vi "test8-UserLog_Queue.vi"(8 "error in (no error)":errorcluster, 11 "TestCase in":refnum<class "testcase-CSMGlobalLog.lvclass">) -> (0 "error out":errorcluster, 3 "TestCase out":refnum<class "testcase-CSMGlobalLog.lvclass">)   [LabVIEW 2017, in "testcase-CSMGlobalLog.lvclass"]
uses:
  testcase-CSMGlobalLog.lvclass
  testcase-CSMGlobalLog.lvclass/testcase-CSMGlobalLog.ctl
  ed57623f-cc02-4141-adee-02d92d4e7552.vi
  src/user.lib/_NEVSTOP/Communicable State Machine(CSM)/_Support/GlobalEvent/GEvt-Generate with Rule Check.vi
  src/user.lib/_NEVSTOP/Communicable State Machine(CSM)/AdvanceAPI/CSM - Convert Error to Argument.vi
  src/user.lib/_NEVSTOP/Communicable State Machine(CSM)/AdvanceAPI/CSM - Make String Arguments Safe.vi
  src/user.lib/_NEVSTOP/Communicable State Machine(CSM)/AdvanceAPI/CSM - Keywords.vi
  src/user.lib/_NEVSTOP/Communicable State Machine(CSM)/_Support/GlobalEvent/Cache-GEvt Refs.vi
  src/user.lib/_NEVSTOP/Communicable State Machine(CSM)/_Support/GlobalEvent/LogFilter/LogFilter - Check.vi
  src/user.lib/_NEVSTOP/Communicable State Machine(CSM)/_Support/GlobalEvent/LogFilter/LogFilter.lvclass
  <vilib>/addons/_JKI Toolkits/VI Tester/TestCase.llb/TestCase.lvclass
  src/user.lib/_NEVSTOP/Communicable State Machine(CSM)/Communicable State Machine.lvlib
  src/user.lib/_NEVSTOP/Communicable State Machine(CSM)/Utility/Periodic String Filter Setting.ctl
  C:/Program Files (x86)/National Instruments/LabVIEW 2017/vi.lib/addons/_JKI Toolkits/VI Tester/TestCase.llb/TestCase.lvclass
panel:
  out "String cache total":string
  out "error out 2":errorcluster
  out "LoopCount":i32
  out "String Cache Each Loop":string
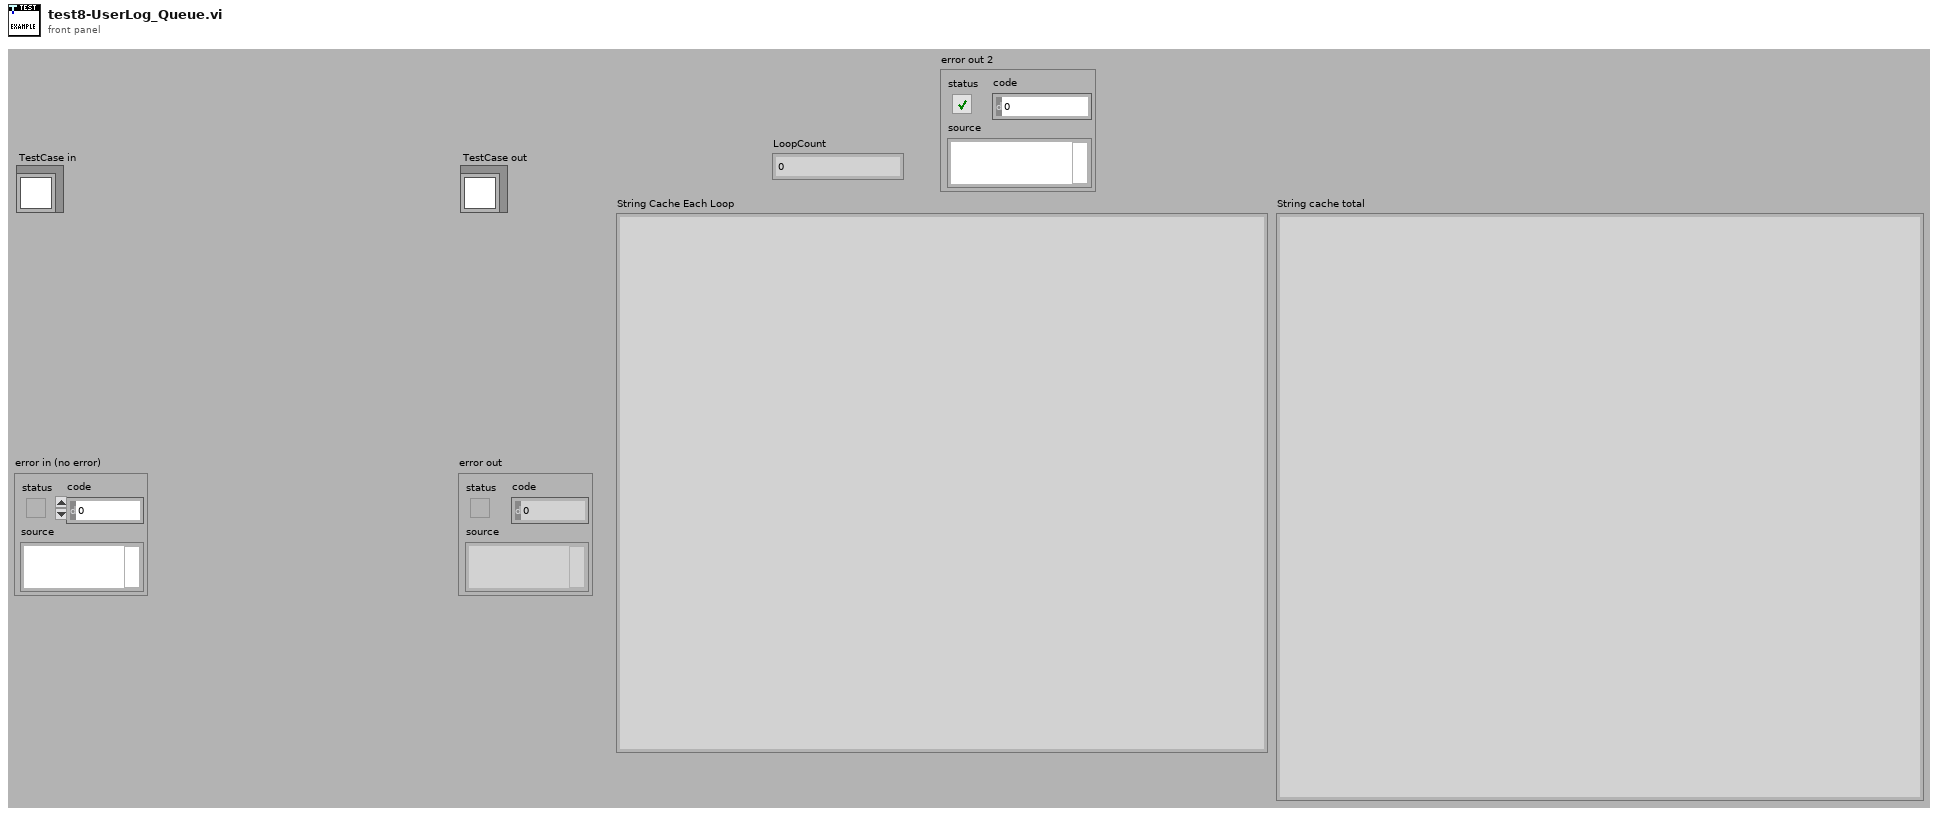
[diagram p1: front panel]
types:
  T1 = typedef "Communicable State Machine.lvlib/Periodic String Filter Setting.ctl" = cluster{"threashold(#/s)":dbl, "Check Peroid(s)":dbl}
  T2 = typedef "Communicable State Machine.lvlib/_CSM_GlobalLog_MSG.ctl" = cluster{"Name (\"\" to Use UUID)":string, "Current State":string, "Arguments":string, "Source Message":T3, "Source Module":string, "Complete(T)/Start(F)":bool, "LogType":T4, "Time Stamp":timestamp}
  T3 = typedef "Communicable State Machine.lvlib/_CSM_Response Source Message.ctl" = cluster{"‘State":string, "’Arguments":string, "’Error":errorcluster}
  T4 = typedef "Communicable State Machine.lvlib/_CSM_GlobalLog_MSG_TYPE.ctl" = enum16{"User Log", "State Change", "Status", "Interrupt", "Register", "Unregister", "Error Log", "Module Created", "Module Destroyed"}
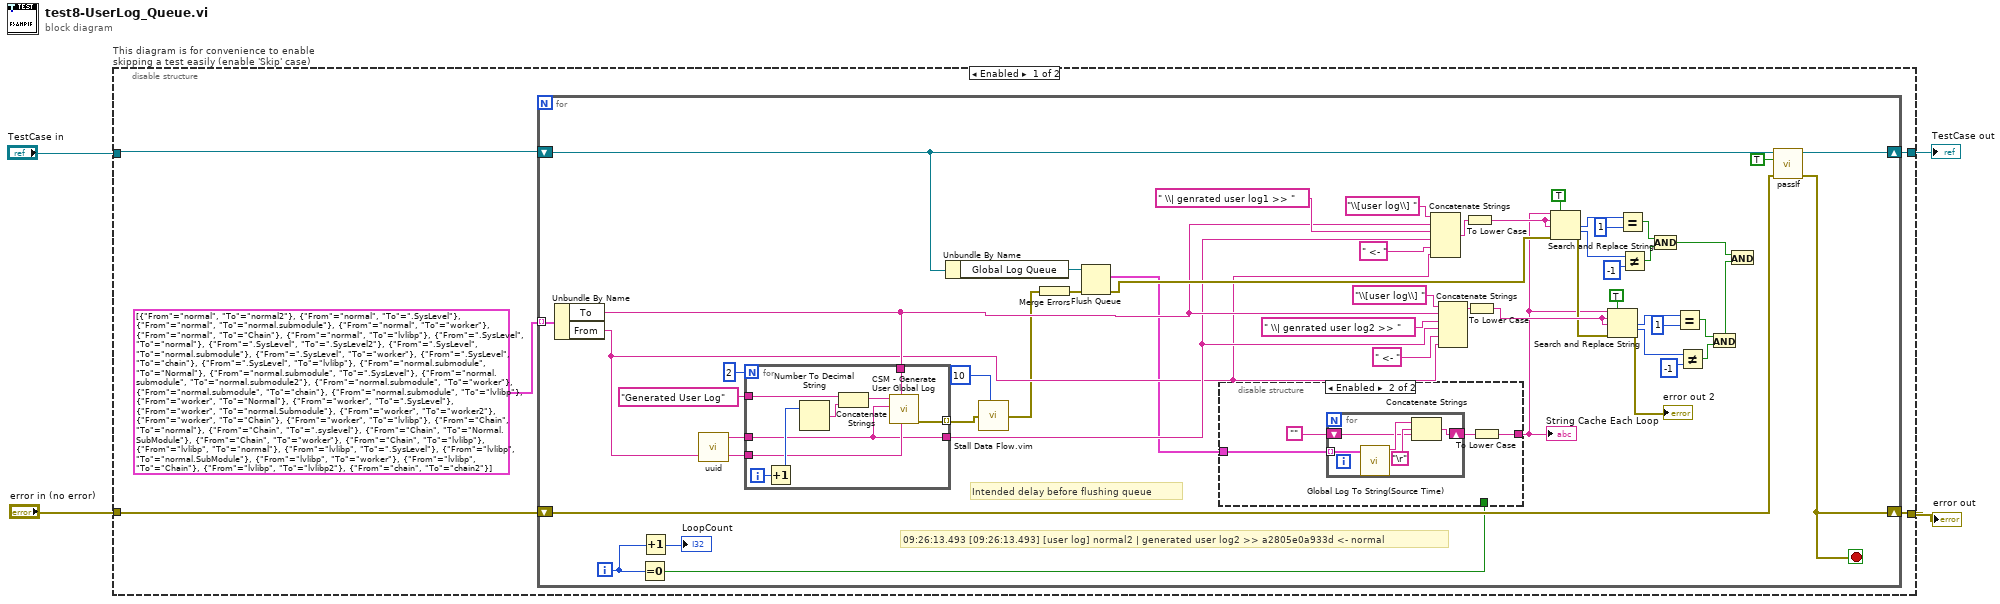
[diagram p0: block diagram]
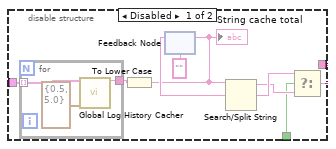
[diagram p2: hidden frame]
diagram:
  n1 = disable-structure "This diagram is for convenience to enable skipping a test easily (enable 'Skip' case)" shown="Enabled" {
    disable-tunnel: "TestCase in" -> [w6 w94]
    disable-tunnel: [w8 w92] -> w1
    disable-tunnel: [w9 w93] -> w3
    disable-tunnel: "error in (no error)" -> [w7 w91]
    frame Enabled {
      n2 = for {
        shift-right: [w35] -> w9
        shift-left: w7 -> [w58]
        shift-right: [w60] -> w8
        shift-left: w6 -> [w34]
        tunnel: cluster{"From":string, "To":string}[] [{"From"="normal", "To"="normal2"}, {"From"="normal", "To"=".SysLevel"}, {"From"="normal", "To"="normal.submodule"}, {"From"="normal", "To"="worker"}, {"From"="normal", "To"="Chain"}, {"From"="normal", "To"="lvlibp"}, {"From"=".SysLevel", "To"="normal"}, {"From"=".SysLevel", "To"=".SysLevel2"}, {"From"=".SysLevel", "To"="normal.submodule"}, {"From"=".SysLevel", "To"="worker"}, {"From"=".SysLevel", "To"="chain"}, {"From"=".SysLevel", "To"="lvlibp"}, {"From"="normal.submodule", "To"="Normal"}, {"From"="normal.submodule", "To"=".SysLevel"}, {"From"="normal.submodule", "To"="normal.submodule2"}, {"From"="normal.submodule", "To"="worker"}, {"From"="normal.submodule", "To"="chain"}, {"From"="normal.submodule", "To"="lvlibp"}, {"From"="worker", "To"="Normal"}, {"From"="worker", "To"=".SysLevel"}, {"From"="worker", "To"="normal.Submodule"}, {"From"="worker", "To"="worker2"}, {"From"="worker", "To"="Chain"}, {"From"="worker", "To"="lvlibp"}, {"From"="Chain", "To"="normal"}, {"From"="Chain", "To"=".syslevel"}, {"From"="Chain", "To"="Normal.SubModule"}, {"From"="Chain", "To"="worker"}, {"From"="Chain", "To"="lvlibp"}, {"From"="lvlibp", "To"="normal"}, {"From"="lvlibp", "To"=".SysLevel"}, {"From"="lvlibp", "To"="normal.SubModule"}, {"From"="lvlibp", "To"="worker"}, {"From"="lvlibp", "To"="Chain"}, {"From"="lvlibp", "To"="lvlibp2"}, {"From"="chain", "To"="chain2"}] -> [w21] mode=indexing
        i -> [w11]
        stop <- w35 stop-if-true
        # "Intended delay before flushing queue"
        # "09:26:13.493 [09:26:13.493] [user log] normal2 | generated user log2 >> a2805e0a933d <- normal"
        n3 = Unbundle By Name(w21) -> ("To"=w20:string, "From"=w17:string)
        n4 = Equal To 0?(x=w11) -> (x = 0?=w10:bool)
        n5 = Increment(x=w11) -> (x+1=→"LoopCount":i32)
        n6 = call "uuid.vi"() -> ("UUID"=w31:string)  [unwired: 11 in]
        n7 = for {
          N: 2 -> [_]
          tunnel: [w90] -> w16 mode=indexing
          tunnel: "Generated User Log" ("Log") -> [w89]
          tunnel: w31 -> [w82]
          tunnel: w20 -> [w84]
          tunnel: w17 -> [w83]
          tunnel: [w82] -> w19
          i -> [w86]
          n8 = Increment(x=w86) -> (x+1=w85:i32)
          n9 = Number To Decimal String(number=w85) -> (decimal integer string=w88:string)  [unwired: 1 in]
          n10 = Concatenate Strings(w89, w88) -> (w87:string)
          n11 = call "CSM - Generate User Global Log.vi"("From Who"=w83, "Place (\"\" to Use VI's Name)"=w84, "Arguments"=w82, "Log"=w87) -> ("error out"=w90:errorcluster)  [unwired: 7 in]
        }
        n12 = Unbundle By Name(w34) -> ("Global Log Queue"=w59:refnum<queue>)
        n13 = call "Stall Data Flow.vim"("value in"=w16, "milliseconds to wait"=u32 10) -> ("value out"=w15:errorcluster[])  [unwired: 1 out]
        n14 = Merge Errors(w15) -> (w30:errorcluster)
        n15 = Flush Queue(queue=w59, error in (no error)=w30) -> (remaining elements=w13:T2[], error out=w40:errorcluster)  [unwired: 1 out]
        n16 = disable-structure shown="Enabled" {
          disable-tunnel: [w63 w73] -> w12
          disable-tunnel: w10 -> [w62 _]
          disable-tunnel: w13 -> [w61 w75]
          frame Disabled {
            n17 = for {
              tunnel: w61 -> [w72] mode=indexing
              tunnel: [w71] -> w69
              n18 = call "Global Log History Cacher.vi"("Global Log Data"=w72, "Settings"=T1 {"threashold(#/s)"=0.5, "Check Peroid(s)"=5.0}) -> ("String Cache"=w71:string)  [unwired: 13 in]
            }
            n19 = To Lower Case(string=w69) -> (all lower case string=w64:string)
            "String cache total" <- w64
            n20 = feedback #1("") -> (w68:string)
            n21 = feedback-in #1(w64) -> ()
            n22 = Search/Split String(string=w64, search string/char (-)=w68) -> (substring before match=w65:string, match + rest of string=w66:string)  [unwired: 1 in, 1 out]
            n23 = Select(t=w66, s=w62, f=w65) -> (s? t:f=w63:string)
          }
          frame Enabled {
            n24 = for {
              tunnel: w75 -> [w81] mode=indexing
              shift-right: [w77] -> w74
              shift-left: "" -> [w78]
              n25 = call "Global Log To String(Source Time).vi"("Log"=w81) -> ("Log String"=w80:string)  [unwired: 9 in]
              n26 = Concatenate Strings(w80, "\r", w78) -> (w77:string)
            }
            n27 = To Lower Case(string=w74) -> (all lower case string=w73:string)
          }
        }
        "String Cache Each Loop" <- w12
        n28 = Concatenate Strings("\\[user log\\] " ("regular expression"), w20, " \\| genrated user log1 >> " ("string"), w19, " <- " ("string"), w17) -> (w25:string)
        n29 = Concatenate Strings("\\[user log\\] " ("regular expression"), w20, " \\| genrated user log2 >> " ("string"), w19, " <- " ("string"), w17) -> (w27:string)
        n30 = To Lower Case(string=w25) -> (all lower case string=w55:string)
        n31 = To Lower Case(string=w27) -> (all lower case string=w43:string)
        n32 = Search and Replace String(replace all?=TRUE ("replace all? (F)"), input string=w12, search string=w55, replace string=w55, error in=w40) -> (number of replacements=w54:i32, offset past replacement=w53:i32, error out=w42:errorcluster)  [unwired: 3 in, 1 out]
        n33 = Search and Replace String(replace all?=TRUE ("replace all? (F)"), input string=w12, search string=w43, replace string=w43, error in=w42) -> (number of replacements=w45:i32, offset past replacement=w46:i32, error out=→"error out 2":errorcluster)  [unwired: 3 in, 1 out]
        n34 = Equal?(x=w54, y=1) -> (x = y?=w51:bool)
        n35 = Not Equal?(x=w53, y=-1) -> (x != y?=w50:bool)
        n36 = And(x=w51, y=w50) -> (x .and. y?=w36:bool)
        n37 = Equal?(x=w45, y=1) -> (x = y?=w48:bool)
        n38 = Not Equal?(x=w46, y=-1) -> (x != y?=w49:bool)
        n39 = And(x=w48, y=w49) -> (x .and. y?=w41:bool)
        n40 = And(x=w36, y=w41) -> ()  [unwired: 1 out]
        n41 = call-dynamic "passIf.vi"("error in (no error)"=w58, "pass"=TRUE, "TestCase in"=w34) -> ("error out"=w35:errorcluster, "TestCase out"=w60:refnum<class "testcase-CSMGlobalLog.lvclass">)  [unwired: 7 in]
      }
    }
    frame Disabled {
      # "skip test result while test is under development"
      n42 = call <vilib>:"skip.vi"("error in (no error)"=w91, "TestCase in"=w94) -> ("error out"=w93:errorcluster, "TestCase out"=w92:refnum<class "testcase-CSMGlobalLog.lvclass">)  [unwired: 8 in]
    }
  }
  "error out" <- w3
  "TestCase out" <- w1
